vi "Handle Events.vi"(8 "error in (no error)":errorcluster, 11 "VIEventHandler":refnum<class "VIEventHandler.lvclass">) -> ()   [LabVIEW 2019, in "ActorEvents.lvlib" / "VIEventHandler.lvclass"]
uses:
  <vilib>/gpm_packages/@cs/mva-viewable/Source/ActorEvents/EventHandler/VIEventHandler/VIEventHandler.lvclass
  C:/Program Files/National Instruments/LabVIEW 2019/vi.lib/gpm_packages/@cs/mva-viewable/Source/ActorEvents/IEventHandler/IEventHandler.lvclass
  <vilib>/gpm_packages/@cs/mva-viewable/Source/ActorEvents/EventHandler/VIEventHandler/VIEventHandler.lvclass/VIEventHandler.ctl
  <vilib>/gpm_packages/@cs/mva-viewable/Source/ActorEvents/IEventHandler/IEventHandler.lvclass/IEventHandler.ctl
  <vilib>/ActorFramework/Message Enqueuer/Message Enqueuer.lvclass/Message Enqueuer.ctl
  <vilib>/event_ctls.llb/lveventtype.ctl
  <vilib>/gpm_packages/@cs/mva-viewable/Source/ActorEvents/IEventAggregator Messages/MenuSelectionMsg/MenuSelectionMsg.lvclass/MenuSelectionMsg.ctl
  <vilib>/gpm_packages/@cs/mva-viewable/Source/ActorEvents/IEventAggregator Messages/EventDataMessage/EventDataMessage.lvclass/EventDataMessage.ctl
  <vilib>/gpm_packages/@cs/mva-viewable/Source/ActorEvents/IEventAggregator Messages/EventDataMessage/Read Discarded.vi
  <vilib>/gpm_packages/@cs/mva-viewable/Source/ActorEvents/IEventHandler/Accessors/Read Timeout [ms].vi
  <vilib>/gpm_packages/@cs/mva-viewable/Source/ActorEvents/IEventHandler/Accessors/Read Event Filter.vi
  <vilib>/gpm_packages/@cs/mva-viewable/Source/ActorEvents/IEventHandler/Accessors/Read EventAggregator Enqueuer.vi
  <vilib>/gpm_packages/@cs/mva-viewable/Source/ActorEvents/IEventHandler/Accessors/Read Timeout Message.vi
  <vilib>/gpm_packages/@cs/mva-viewable/Source/ActorEvents/IEventHandler/Accessors/Read Timeout Message Priority.vi
  <vilib>/gpm_packages/@cs/mva-viewable/Source/ActorEvents/IEventAggregator Messages/EventDataMessage/Send Event Data Message.vi
  <vilib>/Utility/error.llb/Clear Errors.vi
  <vilib>/gpm_packages/@cs/mva-viewable/Source/ActorEvents/IEventAggregator Messages/MenuSelectionMsg/MenuSelectionMsg.lvclass
  C:/Program Files/National Instruments/LabVIEW 2019/vi.lib/gpm_packages/@cs/mva-viewable/Source/ActorEvents/IEventAggregator Messages/EventDataMessage/EventDataMessage.lvclass
  <vilib>/gpm_packages/@cs/mva-viewable/Source/ActorEvents/IEventAggregator Messages/EventDataMessage/EventDataMessage.lvclass
  C:/Program Files/National Instruments/LabVIEW 2019/vi.lib/ActorFramework/Message/Message.lvclass
  <vilib>/gpm_packages/@cs/mva-viewable/Source/ActorEvents/IEventAggregator Messages/PanelCloseMsg/PanelCloseMsg.lvclass
  <vilib>/ActorFramework/Message Priority Queue/Priority Enqueue.vi
  <vilib>/gpm_packages/@cs/mva-viewable/Source/ActorEvents/IEventFilter/IEventFilter.lvclass
  <vilib>/ActorFramework/Message Enqueuer/Message Enqueuer.lvclass
  <vilib>/ActorFramework/Message/Message.lvclass
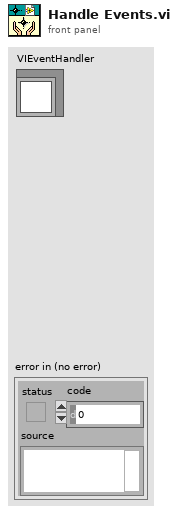
[diagram p1: front panel]
types:
  T1 = typedef "ActorEvents.lvlib/IEventFilter.lvclass/EventFilter Reference.ctl" = refnum<data-value>
  T2 = typedef "Actor Framework.lvlib/Message Enqueuer.lvclass/Message Priority.ctl" = enum16{"Low", "Normal", "High"}
  T3 = typedef "lveventtype.ctl" = enum32{"Null", "Timeout", "Annotation Menu Selection", "Annotation Menu Selection?", "App Instance Close", "App Instance Close?", "Autoscale Range Change", "Bookmark Info Change", "Cell Edit", "Cell Edit?", "Cursor Grab", "Cursor Grab?", "Cursor Menu Selection", "Cursor Menu Selection?", "Cursor Move", "Cursor Release", "Data Change", "Direction Change", "Display State Change", "Drag Ended", "Drag Enter", "Drag Leave", "Drag Over", "Drag Source Update", "Drag Starting", "Drag Starting?", "Drop", "Exec State Change", "Key Down", "Key Down?", "Key Repeat", "Key Repeat?", "Key Up", "Listbox Double Click", "Menu Activation?", "Menu Selection (App)", "Menu Selection? (App)", "Menu Selection (User)", "Mouse Down", "Mouse Down?", "Mouse Enter", "Mouse Leave", "Mouse Move", "Mouse Up", "Mouse Wheel", "NI Security User Change (App)", "Pane Size", "Panel Close", "Panel Close?", "Panel Resize", "Plot Attribute Change", "Scale Range Change", "Shortcut Menu Activation?", "Shortcut Menu Selection (App)", "Shortcut Menu Selection? (App)", "Shortcut Menu Selection (User)", "Tree Double Click", "Tree Drag", "Tree Drag?", "Tree Drop", "Tree Drop?", "Tree Item Close", "Tree Item Close?", "Tree Item Open", "Tree Item Open?", "User Event", "Value Change"}
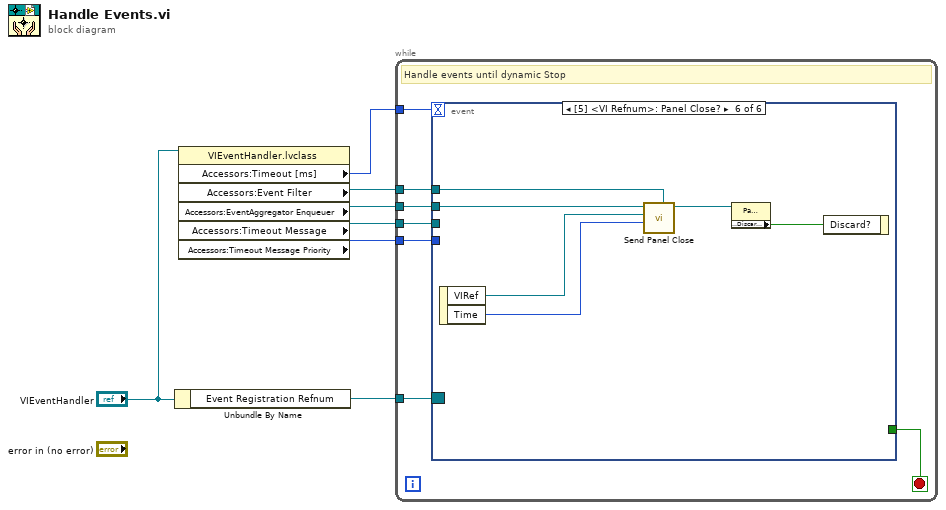
[diagram p0: block diagram]
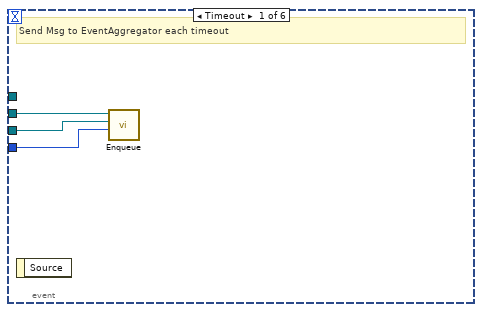
[diagram p2: hidden frame]
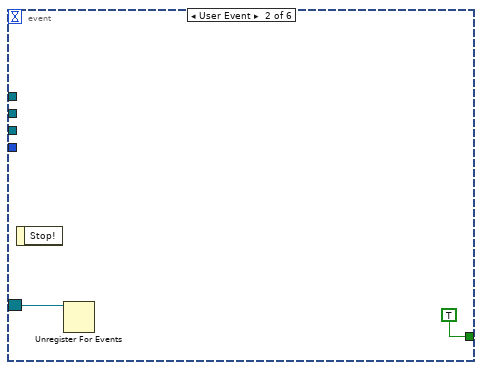
[diagram p3: hidden frame]
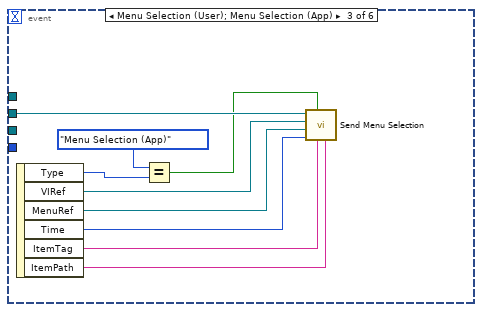
[diagram p4: hidden frame]
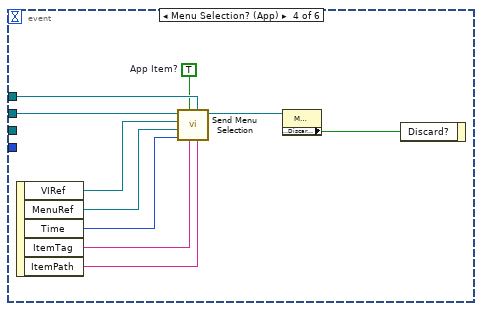
[diagram p5: hidden frame]
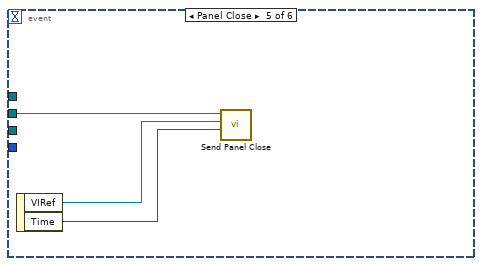
[diagram p6: hidden frame]
diagram:
  n1 = Unbundle By Name("VIEventHandler") -> ("Event Registration Refnum"=w7:refnum<event-registration>)
  n2 = property class="VIEventHandler.lvclass"(reference="VIEventHandler") -> ("Accessors:Timeout [ms]"=w5:i32, "Accessors:Event Filter"=w1:T1, "Accessors:EventAggregator Enqueuer"=w4:refnum<class "Message Enqueuer.lvclass">, "Accessors:Timeout Message"=w3:refnum<class "Message.lvclass">, "Accessors:Timeout Message Priority"=w2:T2)  [unwired: 1 in, 2 out]
  n3 = while {
    tunnel: w7 -> [w14]
    tunnel: w4 -> [w12]
    tunnel: w3 -> [w11]
    tunnel: w2 -> [w10]
    tunnel: w5 -> [w9]
    tunnel: w1 -> [w8]
    stop <- w13 stop-if-true
    # "Handle events until dynamic Stop"
    n4 = event shown="[5] <VI Refnum>: Panel Close?" {
      selector: w14 -> [_ w19 _ _ _ _]
      dyn-events: _ -> [_ _ _ _ _ _]
      timeout: w9 -> [_ _ _ _ _ _]
      tunnel: [_ TRUE ("Stop!") _ _ _ _] -> w13
      tunnel: w12 -> [w17 _ w28 w38 w41 w47]
      tunnel: w11 -> [w16 _ _ _ _ _]
      tunnel: w10 -> [w15 _ _ _ _ _]
      tunnel: w8 -> [_ _ _ w32 _ w43]
      event Timeout {
        # "Send Msg to EventAggregator each timeout"
        n5 = event-data() -> ()  [unwired: 1 in, 1 out]
        n6 = call <vilib>:"Enqueue.vi"("Message Priority (Normal)"=w15, "Message"=w16, "Message Enqueuer in"=w17) -> ()  [unwired: 7 in, 2 out]
      }
      event User Event {
        n7 = event-data() -> ()  [unwired: 1 in, 1 out]
        n8 = Unregister For Events(event registration refnum=w19) -> ()  [unwired: 1 in, 1 out]
      }
      event Menu Selection (User); Menu Selection (App) {
        n9 = event-data() -> ("Type"=w22:T3, "VIRef"=w23:refnum<vi>, "MenuRef"=w24:refnum<k9>, "Time"=w25:u32, "ItemTag"=w27:string, "ItemPath"=w26:string)  [unwired: 1 in]
        n10 = Equal?(x=lveventtype."Menu Selection (App)", y=w22) -> (x = y?=w21:bool)
        n11 = call <vilib>:"Send Menu Selection.vi"("Item Path"=w26, "Item Tag"=w27, "App Item?"=w21, "Time"=w25, "MenuRef"=w24, "VI Refnum"=w23, "Message Enqueuer in"=w28) -> ()  [unwired: 3 in, 2 out]
      }
      event Menu Selection? (App) {
        w31 = TRUE  # App Item?
        n12 = event-data() -> ("VIRef"=w33:refnum<vi>, "MenuRef"=w34:refnum<k9>, "Time"=w35:u32, "ItemTag"=w37:string, "ItemPath"=w36:string)  [unwired: 1 in]
        n13 = call <vilib>:"Send Menu Selection.vi"("Item Path"=w36, "EventFilter Reference"=w32, "Item Tag"=w37, "App Item?"=w31, "Time"=w35, "MenuRef"=w34, "VI Refnum"=w33, "Message Enqueuer in"=w38) -> ("Filtered EventDataMessage"=w30:refnum<class "MenuSelectionMsg.lvclass">)  [unwired: 2 in, 1 out]
        n14 = property class="MenuSelectionMsg.lvclass"(reference=w30) -> ("Accessors:Discarded?"=w29:bool)  [unwired: 1 in, 2 out]
        n15 = event-data("Discard?"=w29) -> ()  [unwired: 1 in, 1 out]
      }
      event Panel Close {
        n16 = event-data() -> ("VIRef"=w40:refnum<vi>, "Time"=w39:u32)  [unwired: 1 in]
        n17 = call <vilib>:"Send Panel Close.vi"("Time"=w39, "VI Refnum"=w40, "Message Enqueuer in"=w41) -> ()  [unwired: 7 in, 2 out]
      }
      event Panel Close? {
        n18 = event-data() -> ("VIRef"=w46:refnum<vi>, "Time"=w45:u32)  [unwired: 1 in]
        n19 = call <vilib>:"Send Panel Close.vi"("EventFilter Reference"=w43, "Time"=w45, "VI Refnum"=w46, "Message Enqueuer in"=w47) -> ("Filtered EventDataMessage"=w44:refnum<class "PanelCloseMsg.lvclass">)  [unwired: 6 in, 1 out]
        n20 = property class="PanelCloseMsg.lvclass"(reference=w44) -> ("Accessors:Discarded?"=w42:bool)  [unwired: 1 in, 2 out]
        n21 = event-data("Discard?"=w42) -> ()  [unwired: 1 in, 1 out]
      }
    }
  }
